vi "Clear Logger.vi"(8 "error in (no error)":errorcluster, 11 "Logger Normal in":refnum<class "Logger Normal.lvclass">) -> (0 "error out":errorcluster, 3 "Logger Normal out":refnum<class "Logger Normal.lvclass">)   [LabVIEW 2020, in "Logger Normal.lvlib" / "Logger Normal.lvclass"]
uses:
  Logger Normal.lvclass
  Logger Normal Messages/Clear Msg/Clear Msg.lvclass
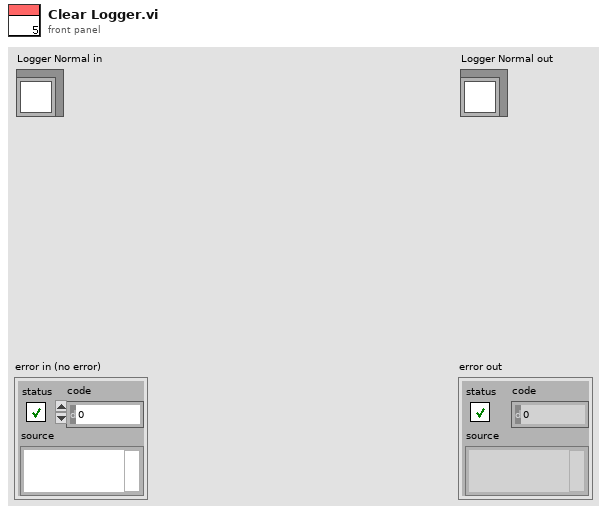
[diagram p1: front panel]
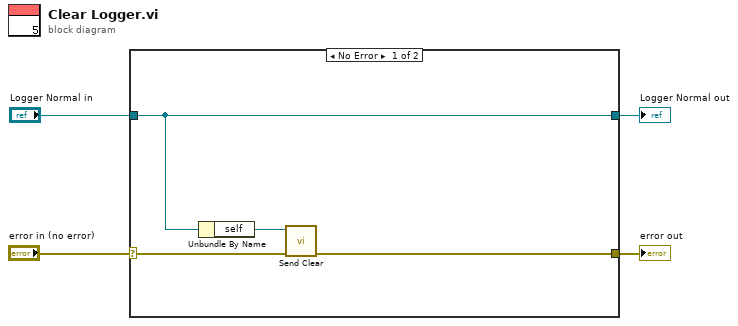
[diagram p0: block diagram]
diagram:
  n1 = case shown="No Error" "error in (no error)" {
    selector: "error in (no error)" -> [w7 w10]
    tunnel: "Logger Normal in" -> [w8 w9]
    tunnel: [w6 w10] -> w2
    tunnel: [w8 w9] -> w1
    frame No Error {
      n2 = Unbundle By Name(w8) -> ("self"=w5:refnum<class "Message Enqueuer.lvclass">)
      n3 = call "Send Clear.vi"("error in (no error)"=w7, "Message Enqueuer"=w5) -> ("error out"=w6:errorcluster)  [unwired: 8 in, 1 out]
    }
    frame Error {
    }
  }
  "error out" <- w2
  "Logger Normal out" <- w1
